vi "Read template.vi"() -> ()   [LabVIEW 2012]
doc: "This VI shows how to use Network Streams to read data generated from a another process."
uses:
  Datatype B.ctl
panel:
  in  "stop":bool
  out "Data B read":T1
  in  "Data B writer endpoint URL":string="//localhost/Data B Writer Name"
  # "Open \n     Read write template.vi\nfor instructions on how to use this template."
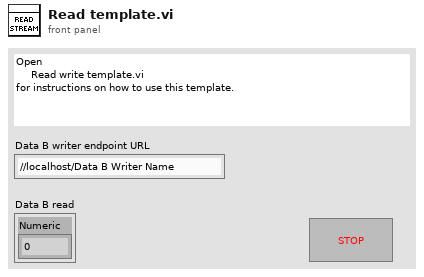
[diagram p1: front panel]
types:
  T1 = typedef "Datatype B.ctl" = cluster{"Numeric":dbl}
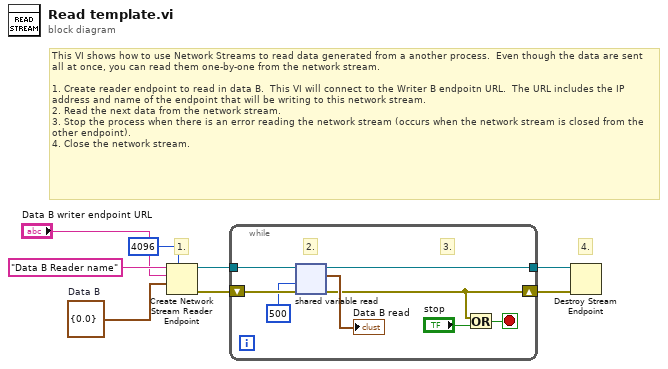
[diagram p0: block diagram]
diagram:
  w2 = T1 {"Numeric"=0.0}  # Data B
  # "4."
  # "1."
  # "This VI shows how to use Network Streams to read data generated from a another process.  Even though the data are sent all at once, you can read them one-by-one from the network stream.\n\n1. Create reader endpoint to read in data B.  This VI will connect to the Writer B endpoitn URL.  The URL includes the IP address and name of the endpoint that will be writing to this network stream.\n2. Read the next data from the network stream.\n3. Stop the process when there is an error reading the network stream (occurs when the network stream is closed from the other endpoint).\n4. Close the network stream."
  n1 = Create Network Stream Reader Endpoint(7:4096 ("reader buffer size"), 9:w2, 10:"Data B writer endpoint URL", 11:"Data B Reader name" ("reader name")) -> (0:w5:errorcluster, 3:w6:refnum<k21>)  [unwired: 3 in]
  n2 = while {
    tunnel: w6 -> [w16]
    tunnel: [w14] -> w4
    shift-right: [w10] -> w3
    shift-left: w5 -> [w15]
    stop <- w9 stop-if-true
    # "3."
    # "2."
    n3 = shared-variable-read(w16, w15, 500 ("timeout ms (-1)")) -> (w14:refnum<k21>, w10:errorcluster, →"Data B read":T1)  [unwired: 1 out]
    n4 = Or(x=w10, y="stop") -> (x .or. y?=w9:bool)
  }
  n5 = Destroy Stream Endpoint(8:w3, 11:w4) -> ()  [unwired: 1 out]
